vi "Infinitesimal Displacement.vi"(4 "dt":dbl, 5 "[xc yc phic]":dbl[](array[numeric]), 6 "[Cx Cy Cz]":dbl[](array[numeric]), 7 "[Fux Fuy Tuz]":dbl[](array[numeric])) -> (0 "Rd":T1, 1 "Rc":T1, 2 "[xd yd phid]":dbl[](array[numeric])=[-0.1873242819365118, 0.0, 0.0], 3 "[xc yc zc]":dbl[](array[numeric]))   [LabVIEW 2017]
uses:
  <vilib>/Analysis/Matrix/Datatypes/RealMatrix.ctl
  <vilib>/Analysis/_algsub.llb/Real Vector Norm.vi
  <vilib>/Analysis/baseanly.llb/Real A x B.vi
  <vilib>/Analysis/baseanly.llb/A x Vector.vi
  <vilib>/Analysis/baseanly.llb/Outer Product.vi
  <vilib>/Analysis/baseanly.llb/Real Outer Product.vi
  <vilib>/robotics/Kinematics/Create Lie Group Matrix.vi
  <vilib>/Analysis/7linalg.llb/Create Special Matrix.vi
  <vilib>/Analysis/7linalg.llb/Create Special Real Matrix.vi
  <vilib>/Analysis/Matrix/Numeric/Multiply/Multiply.vi
  <vilib>/Analysis/Matrix/Numeric/Multiply/Multiply - RM,R.vi
  <vilib>/Analysis/Matrix/Numeric/Multiply/Multiply - R,RM.vi
  <vilib>/Analysis/Matrix/Numeric/Add/Add.vi
  <vilib>/Analysis/Matrix/Numeric/Add/Add - RM,RM.vi
  <vilib>/Analysis/NI_AALPro.lvlib
  <vilib>/Analysis/NI_AALBase.lvlib
  <vilib>/robotics/Kinematics/NI_Kinematics.lvlib
  <vilib>/Analysis/Matrix/NI_Matrix.lvlib
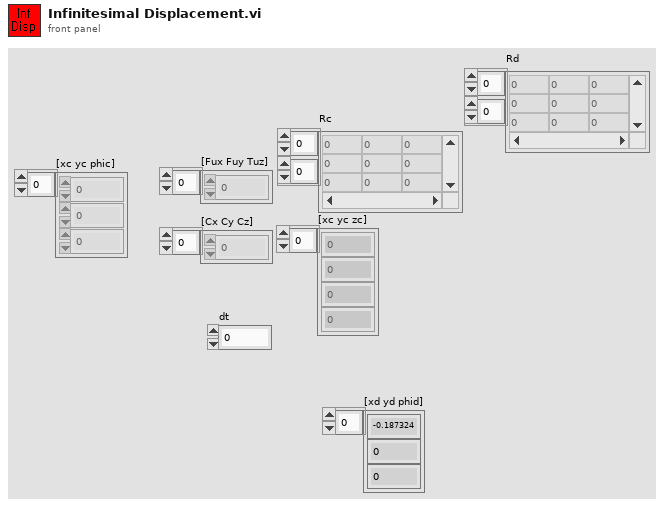
[diagram p1: front panel]
types:
  T1 = typedef "NI_Matrix.lvlib/RealMatrix.ctl" = dbl[][]
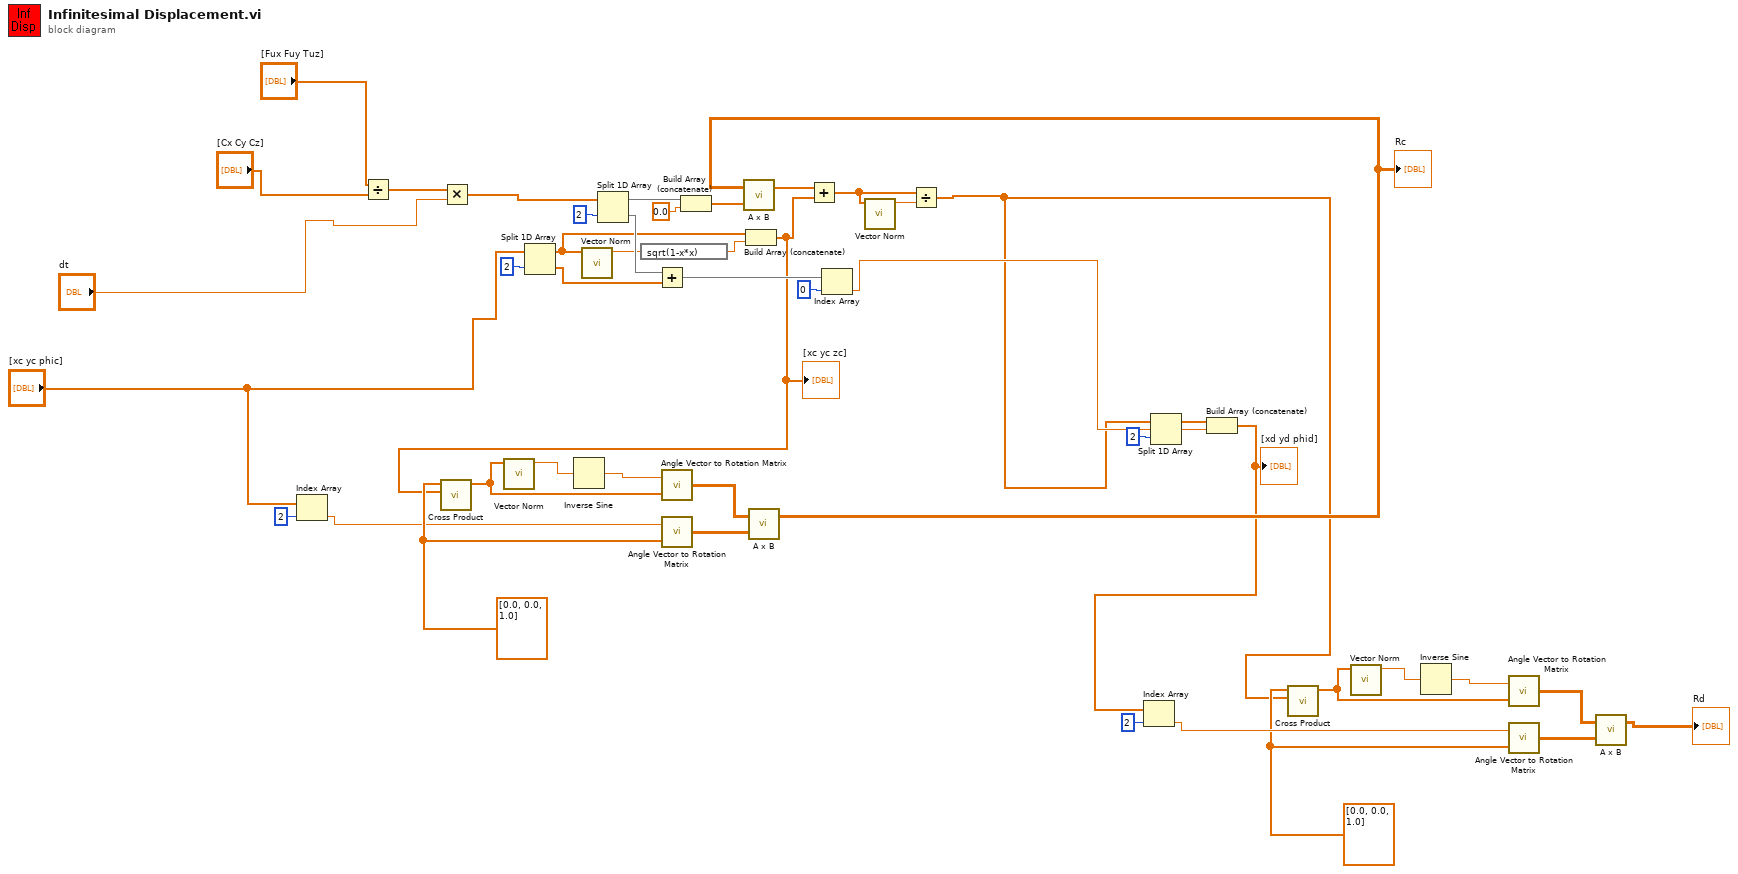
[diagram p0: block diagram]
diagram:
  w7 = dbl[] [0.0, 0.0, 1.0] ("A Vector")
  w21 = dbl[] [0.0, 0.0, 1.0] ("A Vector")
  n1 = Index Array(array="[xc yc phic]", index=2) -> (element=w16:dbl)
  n2 = Divide(x="[Fux Fuy Tuz]", y="[Cx Cy Cz]") -> (x/y=w45:dbl[])
  n3 = Multiply(x=w45, y="dt") -> (x*y=w12:dbl[])
  n4 = Split 1D Array(array="[xc yc phic]", index=2) -> (first subarray=w33:dbl[], second subarray=w39:dbl[])
  n5 = call-poly <vilib>:"Vector Norm.vi"("Input Vector"=w33) -> ("norm"=w34:dbl)  [unwired: 9 in, 1 out]
  n6 = Split 1D Array(array=w12, index=2) -> (first subarray=w37:dbl[], second subarray=w40:dbl[])
  n7 = expression code="sqrt(1-x*x)"(w34) -> (w32:dbl)
  n8 = Add(x=w40, y=w39) -> (x+y=w29:dbl[])
  n9 = call <vilib>:"Angle Vector to Rotation Matrix.vi"("vector"=w21, "angle"=w16) -> ("rotation matrix"=w19:T1)
  n10 = Build Array (concatenate)(w37, 0.0) -> (w35:dbl[])
  n11 = Build Array (concatenate)(w33, w32) -> (w15:dbl[])
  "[xc yc zc]" <- w15
  n12 = call <vilib>:"Cross Product.vi"("B Vector"=w15, "A Vector"=w21) -> ("Cross Product"=w23:dbl[])  [unwired: 8 in, 1 out]
  n13 = call-poly <vilib>:"Vector Norm.vi"("Input Vector"=w23) -> ("norm"=w24:dbl)  [unwired: 9 in, 1 out]
  n14 = Inverse Sine(1:w24) -> (0:w22:dbl)
  n15 = call <vilib>:"Angle Vector to Rotation Matrix.vi"("vector"=w23, "angle"=w22) -> ("rotation matrix"=w20:T1)
  n16 = call-poly <vilib>:"A x B.vi"("B"=w19, "A"=w20) -> ("A x B"=w14:T1)  [unwired: 1 out]
  "Rc" <- w14
  n17 = call-poly <vilib>:"A x B.vi"("Vector"=w35, "A"=w14) -> ("A x Vector"=w38:dbl[])  [unwired: 1 out]
  n18 = Add(x=w38, y=w15) -> (x+y=w41:dbl[])
  n19 = Index Array(array=w29, index=0) -> (element=w27:dbl)
  n20 = call-poly <vilib>:"Vector Norm.vi"("Input Vector"=w41) -> ("norm"=w42:dbl)  [unwired: 9 in, 1 out]
  n21 = Divide(x=w41, y=w42) -> (x/y=w2:dbl[])
  n22 = Split 1D Array(array=w2, index=2) -> (first subarray=w30:dbl[])  [unwired: 1 out]
  n23 = Build Array (concatenate)(w30, w27) -> (w3:dbl[])
  "[xd yd phid]" <- w3
  n24 = Index Array(array=w3, index=2) -> (element=w11:dbl)
  n25 = call <vilib>:"Cross Product.vi"("B Vector"=w2, "A Vector"=w7) -> ("Cross Product"=w5:dbl[])  [unwired: 8 in, 1 out]
  n26 = call-poly <vilib>:"Vector Norm.vi"("Input Vector"=w5) -> ("norm"=w4:dbl)  [unwired: 9 in, 1 out]
  n27 = Inverse Sine(1:w4) -> (0:w6:dbl)
  n28 = call <vilib>:"Angle Vector to Rotation Matrix.vi"("vector"=w5, "angle"=w6) -> ("rotation matrix"=w8:T1)
  n29 = call <vilib>:"Angle Vector to Rotation Matrix.vi"("vector"=w7, "angle"=w11) -> ("rotation matrix"=w9:T1)
  n30 = call-poly <vilib>:"A x B.vi"("B"=w9, "A"=w8) -> ("A x B"=→"Rd":T1)  [unwired: 1 out]
